vi "Next Step.vi"(8 "error in (no error)":errorcluster, 11 "Wavelength iHR320 in":refnum<class "Wavelength iHR320.lvclass">) -> (0 "error out":errorcluster, 1 "Current Step #":u32, 2 "Current WL":dbl, 3 "Wavelength iHR320 out":refnum<class "Wavelength iHR320.lvclass">)   [LabVIEW 2009, in "Wavelength iHR320.lvclass"]
doc: "(Dynamic) Move to the next preconfigured step of this Scanner, and return the current position (actual, not intended) of this Scanner. Increment the step counter by one."
uses:
  Wavelength iHR320.lvclass
  Scanner/Scanner.lvclass
  Wavelength iHR320.lvclass/Wavelength iHR320.ctl
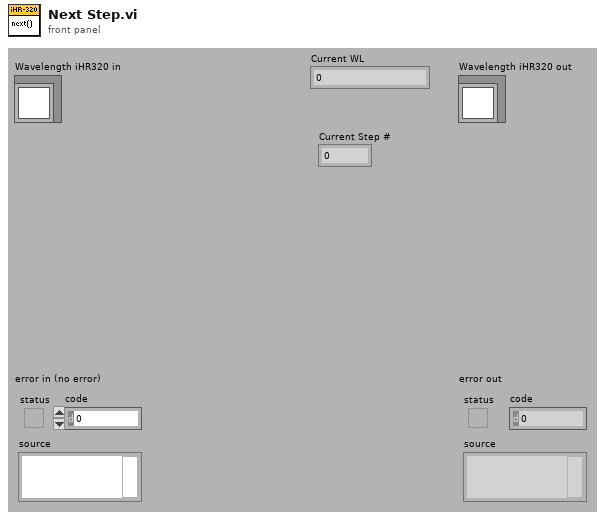
[diagram p1: front panel]
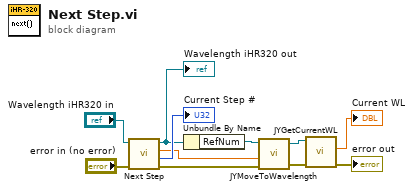
[diagram p0: block diagram]
diagram:
  n1 = call-parent "Next Step.vi"("error in (no error)"="error in (no error)", "Scanner in"="Wavelength iHR320 in") -> ("error out"=w2:errorcluster, "Current Step"=→"Current Step #":u32, "Current Position"=w8:dbl, "Scanner out"=w3:refnum<class "Wavelength iHR320.lvclass">)  [unwired: 6 in]
  "Wavelength iHR320 out" <- w3
  n2 = Unbundle By Name(w3) -> ("RefNum"=w4:refnum<k7>)
  n3 = call "JYMoveToWavelength.vi"("error in (no error)"=w2, "Target WL"=w8, "RefNum In"=w4) -> ("error out"=w6:errorcluster, "Refnum Out"=w7:refnum<k7>)  [unwired: 1 in, 1 out]
  n4 = call "JYGetCurrentWL.vi"("error in (no error)"=w6, "JYMONOLib.IJYMonoReqd In"=w7) -> ("error out"=→"error out":errorcluster, "Current WL"=→"Current WL":dbl)  [unwired: 6 in, 2 out]
